vi "Terminate.vi"(8 "error in (no error)":errorcluster, 11 "Sequencer Core in":refnum<class "Sequencer Core.lvclass">) -> (0 "error out":errorcluster, 3 "Sequencer Core out":refnum<class "Sequencer Core.lvclass">)   [LabVIEW 2020, in "Sequencer.lvlib" / "Sequencer Core.lvclass"]
doc: "Terminate the Message Priority Queue and the Interrupt Notifier and then call the Stop Core method."
uses:
  Sequencer Core.lvclass
  Sequencer Core.lvclass/Sequencer Core.ctl
  Message Priority Queue/Message Priority Queue.lvclass
  PPL/HDH.Data.Generic.lvlibp/Synchronization/Notifier/Notifier.lvclass
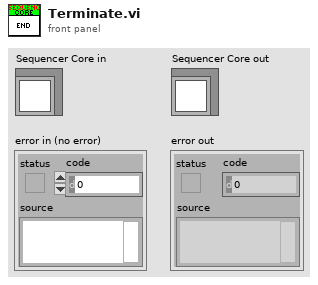
[diagram p1: front panel]
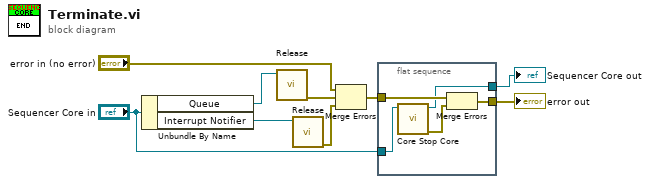
[diagram p0: block diagram]
diagram:
  n1 = Unbundle By Name("Sequencer Core in") -> ("Queue"=w9:refnum<class "Message Priority Queue.lvclass">, "Interrupt Notifier"=w8:refnum<class "Notifier.lvclass">)
  n2 = call "Release.vi"("Priority Queue"=w9) -> ("error out"=w6:errorcluster)  [unwired: 9 in, 1 out]
  n3 = call "Release.vi"("Notifier in"=w8) -> ("error out"=w5:errorcluster)  [unwired: 8 in, 2 out]
  n4 = Merge Errors("error in (no error)", w6, w5) -> (w4:errorcluster)
  n5 = flat-sequence {
    tunnel: w4 -> [w14]
    tunnel: [w12] -> w3
    tunnel: "Sequencer Core in" -> [w11]
    tunnel: [w10] -> w1
    frame #0 {
      n6 = call-dynamic "Core Stop Core.vi"("Sequencer Core in"=w11) -> ("error out"=w13:errorcluster, "Sequencer Core out"=w10:refnum<class "Sequencer Core.lvclass">)  [unwired: 9 in]
      n7 = Merge Errors(w14, w13) -> (w12:errorcluster)
    }
  }
  "error out" <- w3
  "Sequencer Core out" <- w1
